vi "Init.vi"(8 "error in (no error)":errorcluster) -> (0 "error out":errorcluster, 3 "ModbusSp out":refnum<class "ModbusSp.lvclass">)   [LabVIEW 2019, in "ModbusSp.lvclass"]
uses:
  ModbusSp.lvclass
  WriteData.ctl
  ReadData.ctl
  ModbusSp.lvclass/ModbusSp.ctl
  <vilib>/NI/Modbus Library/API/Wrapper/Create TCP Slave.vi
  <vilib>/NI/Modbus Library/API/Wrapper/API Main.lvlib
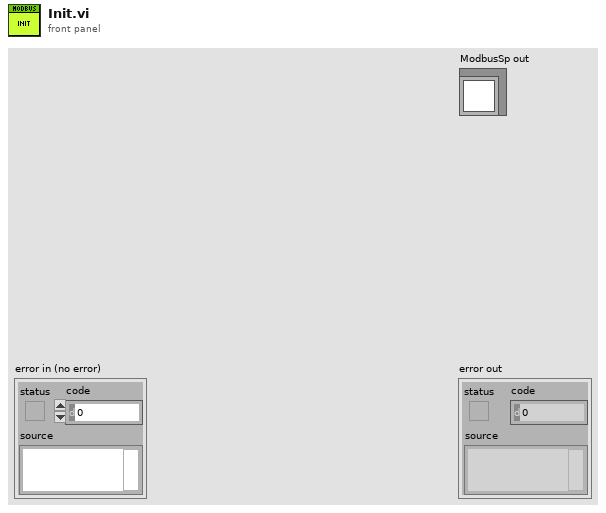
[diagram p1: front panel]
types:
  T1 = typedef "ModbusSp.lvclass/ReadData.ctl" = cluster{"SP":sgl, "Direction":u16, "CMD":u16}
  T2 = typedef "ModbusSp.lvclass/WriteData.ctl" = cluster{"STS":u16, "AI 0":sgl, "AI 1":sgl, "AI 2":sgl, "AI 3":sgl, "AI 4":sgl, "AI 5":sgl, "AI 6":sgl, "AI 7":sgl, "AI 8":sgl, "AI 9":sgl, "AI 10":sgl}
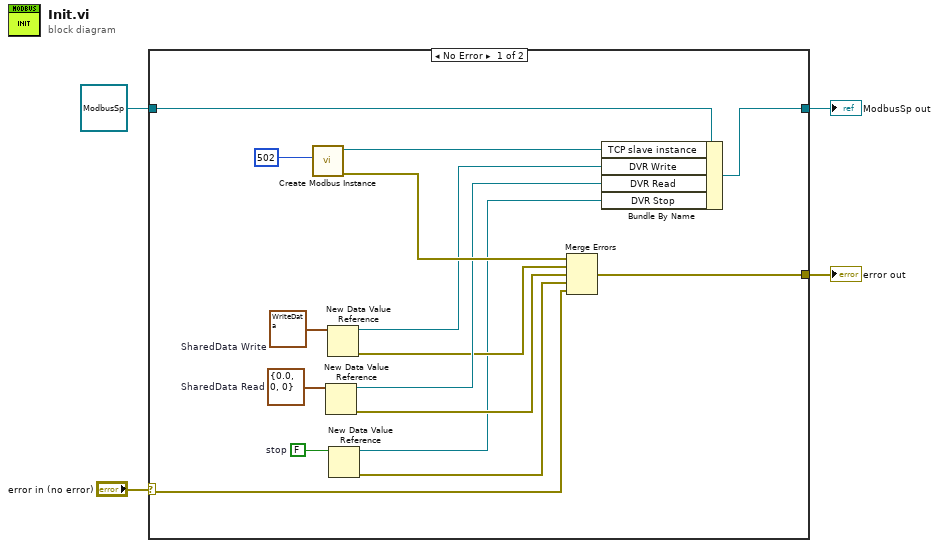
[diagram p0: block diagram]
diagram:
  n1 = case shown="No Error" "error in (no error)" {
    selector: "error in (no error)" -> [w5 w22]
    tunnel: [w11 w22] -> w3
    tunnel: [w17 w21] -> w1
    tunnel: refnum<class "ModbusSp.lvclass"> refnum ("ModbusSp in") -> [w20 w21]
    frame No Error {
      w8 = FALSE  # stop
      w14 = T1 {"SP"=0.0, "Direction"=0, "CMD"=0}  # SharedData Read
      w15 = T2 {"STS"=0, "AI 0"=0.0, "AI 1"=0.0, "AI 2"=0.0, "AI 3"=0.0, "AI 4"=0.0, "AI 5"=0.0, "AI 6"=0.0, "AI 7"=0.0, "AI 8"=0.0, "AI 9"=0.0, "AI 10"=0.0}  # SharedData Write
      n2 = call-poly <vilib>:"Create Modbus Instance.vi"("port (502)"=u16 502) -> ("error out"=w18:errorcluster, "TCP slave instance"=w16:refnum<class "Modbus Slave.lvclass">)  [unwired: 9 in]
      n3 = New Data Value Reference(data value=w14) -> (data value reference=w12:refnum<data-value>, error out=w9:errorcluster)  [unwired: 1 in]
      n4 = New Data Value Reference(data value=w15) -> (data value reference=w13:refnum<data-value>, error out=w10:errorcluster)  [unwired: 1 in]
      n5 = New Data Value Reference(data value=w8) -> (data value reference=w6:refnum<data-value>, error out=w7:errorcluster)  [unwired: 1 in]
      n6 = Merge Errors(w18, w10, w9, w7, w5) -> (w11:errorcluster)
      n7 = Bundle By Name(cluster=w20, "TCP slave instance"=w16, "DVR Write"=w13, "DVR Read"=w12, "DVR Stop"=w6) -> (w17:refnum<class "ModbusSp.lvclass">)
    }
    frame Error {
    }
  }
  "error out" <- w3
  "ModbusSp out" <- w1
